vi "update_data_representation_fullSD.vi"(0 "Commentaires exp":refnum<vi>, 1 "Experiment":T1, 3 "error in (no error)":errorcluster, 4 "# exp":i32, 5 "Experiments groups":refnum<class "Experiments_group.lvclass">[](array[class]), 6 "Group":refnum<vi>) -> (2 "timedelays":dbl[](array[numeric]), 7 "Data":dbl[][](array[numeric]), 8 "error out":errorcluster, 9 "wavelengths":dbl[](array[numeric]))   [LabVIEW 2015]
uses:
  Classes/Experiments_group.lvclass
  controls/mylistboxRef.ctl
  controls/mylistbox.ctl
  Classes/Experiment.lvclass
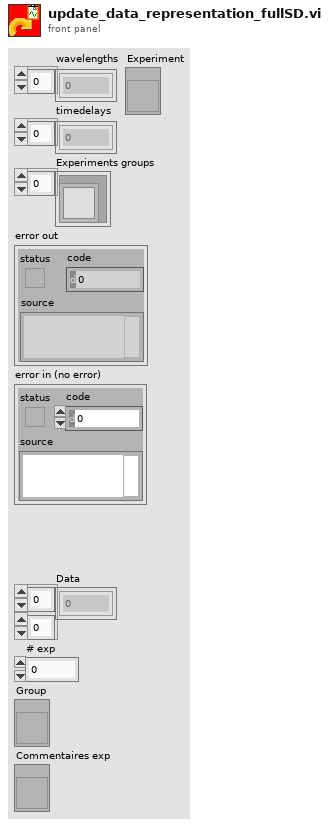
[diagram p1: front panel]
types:
  T1 = typedef "mylistboxRef.ctl" = refnum<vi>
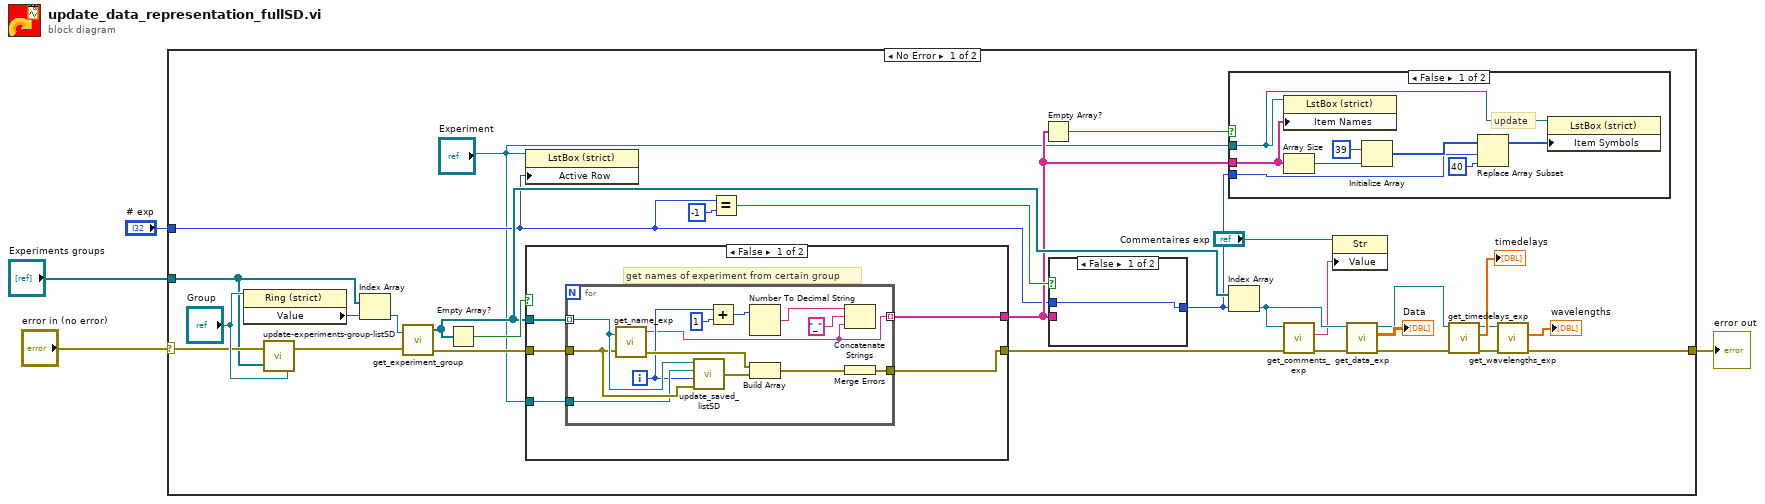
[diagram p0: block diagram]
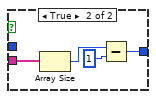
[diagram p2: hidden frame]
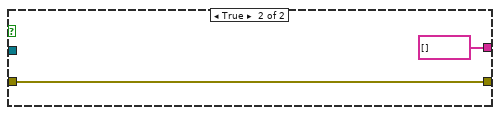
[diagram p3: hidden frame]
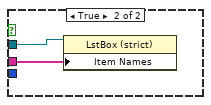
[diagram p4: hidden frame]
diagram:
  n1 = case shown="No Error" "error in (no error)" {
    selector: "error in (no error)" -> [w23 w69]
    tunnel: [w6 w69] -> w3
    tunnel: "Experiments groups" -> [w22 _]
    tunnel: "# exp" -> [w14 _]
    frame No Error {
      n2 = property class="Ring (strict)"(reference="Group") -> ("Value"=w29:u16)  [unwired: 1 in, 2 out]
      n3 = call "update-experiments-group-listSD.vi"("Group"="Group", "Experiments groups"=w22, "error in (no error)"=w23) -> ("error out"=w26:errorcluster)
      n4 = Index Array(array=w22, index=w29) -> (element=w28:refnum<class "Experiments_group.lvclass">)
      n5 = call-dynamic "get_experiment_group.vi"("Experiments_group.lvclass in"=w28, "error in (no error)"=w26) -> ("Experiments"=w20:refnum<class "Experiment.lvclass">[], "error out"=w19:errorcluster)  [unwired: 1 out]
      n6 = Empty Array?(array=w20) -> (empty?=w21:bool)
      n7 = property on="Property Node" class="LstBox (strict)"(reference="Experiment", "Active Row"=w14) -> ()  [unwired: 1 in, 2 out]
      n8 = case shown="False" w21 {
        tunnel: w20 -> [w43 _]
        tunnel: [w42 w58] -> w10
        tunnel: w19 -> [w41 w58]
        tunnel: [w40 string[] []] -> w15
        tunnel: "Experiment" -> [w39 _]
        frame False {
          # "get names of experiment from certain group"
          n9 = for {
            tunnel: w43 -> [w52] mode=indexing
            tunnel: [w45] -> w40 mode=indexing
            tunnel: [w49] -> w42
            tunnel: w41 -> [w48]
            tunnel: w39 -> [w47]
            i -> [w46]
            n10 = call-dynamic "get_name_exp.vi"("Experiment.lvclass in"=w52, "error in (no error)"=w48) -> ("Exp name"=w45:string, "error out"=w51:errorcluster)  [unwired: 1 out]
            n11 = call "update_saved_listSD.vi"("error in (no error)"=w48, "Numeric"=w46, "Experiment"=w47, "Experiment in"=w52) -> ("error out"=w50:errorcluster)
            n12 = Add(x=w46, y=1) -> (x+y=w56:i32)
            n13 = Number To Decimal String(number=w56) -> (decimal integer string=w54:string)  [unwired: 1 in]
            n14 = Build Array(w51, w50) -> (w44:errorcluster[])
            n15 = Concatenate Strings(w54, "_" ("string"), w45) -> ()  [unwired: 1 out]
            n16 = Merge Errors(w44) -> (w49:errorcluster)
          }
        }
        frame True {
        }
      }
      n17 = Equal?(x=w14, y=-1) -> (x = y?=w17:bool)
      n18 = Empty Array?(array=w15) -> (empty?=w33:bool)
      n19 = case shown="False" w17 {
        tunnel: [w34 w36] -> w16
        tunnel: w14 -> [w34 _]
        tunnel: w15 -> [_ w38]
        frame False {
        }
        frame True {
          n20 = Array Size(array=w38) -> (size(s)=w37:i32)
          n21 = Subtract(x=w37, y=1) -> (x-y=w36:i32)
        }
      }
      n22 = case shown="False" w33 {
        tunnel: w15 -> [w61 w68]
        tunnel: "Experiment" -> [w60 w67]
        tunnel: w16 -> [w59 _]
        frame False {
          # "update"
          n23 = property on="Property Node" class="LstBox (strict)"(reference=w60, "Item Names"=w61) -> ()  [unwired: 1 in, 2 out]
          n24 = Array Size(array=w61) -> (size(s)=w62:i32)
          n25 = Initialize Array(39, w62) -> (w64:i32[])
          n26 = Replace Array Subset(array=w64, new element=40 ("new element/subarray"), index=w59) -> (w63:i32[])
          n27 = property on="Property Node" class="LstBox (strict)"(reference=w60, "Item Symbols"=w63) -> ()  [unwired: 1 in, 2 out]
        }
        frame True {
          n28 = property on="Property Node" class="LstBox (strict)"(reference=w67, "Item Names"=w68) -> ()  [unwired: 1 in, 2 out]
        }
      }
      n29 = Index Array(array=w20, index=w16) -> (element=w32:refnum<class "Experiment.lvclass">)
      n30 = call-dynamic "get_comments_exp.vi"("error in (no error)"=w10, "Experiment.lvclass in"=w32) -> ("error out"=w25:errorcluster, "Comments"=w30:string)  [unwired: 7 in, 1 out]
      n31 = property class="Str"(reference="Commentaires exp", "Value"=w30) -> ()  [unwired: 1 in, 2 out]
      n32 = call-dynamic "get_data_exp.vi"("error in (no error)"=w25, "Experiment.lvclass in"=w32) -> ("error out"=w12:errorcluster, "Data"=→"Data":dbl[][], "Experiment.lvclass out"=w13:refnum<class "Experiment.lvclass">)  [unwired: 7 in]
      n33 = call-dynamic "get_timedelays_exp.vi"("error in (no error)"=w12, "Experiment.lvclass in"=w13) -> ("error out"=w7:errorcluster, "timedelays"=→"timedelays":dbl[], "Experiment.lvclass out"=w9:refnum<class "Experiment.lvclass">)  [unwired: 7 in]
      n34 = call-dynamic "get_wavelengths_exp.vi"("error in (no error)"=w7, "Experiment.lvclass in"=w9) -> ("error out"=w6:errorcluster, "wavelengths"=→"wavelengths":dbl[])  [unwired: 7 in, 1 out]
    }
    frame Error {
    }
  }
  "error out" <- w3
